vi "Change Steering Type.vi"(8 "error in (no error)":errorcluster, 10 "steering type":T1 items=["User Defined", "Differential", "Ackermann", "Mecanum"], 11 "dialog info in":T2={"steering frame ref"=refnum, "active wheel indexes"=[], "FP Refs"={"VI Refnum"=refnum, "Menu Ref"=refnum, "Sub Panel"=refnum, "picture"=refnum, "Steering Type"=refnum, "zoom in"=refnum, "zoom out"=refnum, "zoom extents"=refnum, "Wheels"=refnum, "Add Wheel"=refnum, "Remove Wheel"=refnum, "Copy Wheel"=refnum, "Angle Units"=refnum}, "subpanel info"={"subpanel VI refs"=[], "subpanel types"=[], "main to subpanel command events"=[]}, "picture dragging state"={"dragging"=FALSE, "wheel index"=-1, "dragging mode"=enum."translate", "wheel start position"={"x"=0.0, "y"=0.0, "theta"=0.0}, "relative mouse position"={"x"=0.0, "y"=0.0}, "relative mouse init angle (rad)"=0.0}, "picture size (pixels)"={"Width"=500, "Height"=500}, "picture grid"=bytes[0], "click zones group"={"click zones array"=[], "num click zones"=0}, "draw options"={"draw wheel states?"=FALSE, "highlight wheel index"=-1, "pixels per unit"=10.0, "draw forward velocity?"=FALSE, "velocity scale"=1.0}}) -> (0 "error out":errorcluster, 3 "dialog info out":T2={"steering frame ref"=refnum, "active wheel indexes"=[], "FP Refs"={"VI Refnum"=refnum, "Menu Ref"=refnum, "Sub Panel"=refnum, "picture"=refnum, "Steering Type"=refnum, "zoom in"=refnum, "zoom out"=refnum, "zoom extents"=refnum, "Wheels"=refnum, "Add Wheel"=refnum, "Remove Wheel"=refnum, "Copy Wheel"=refnum, "Angle Units"=refnum}, "subpanel info"={"subpanel VI refs"=[], "subpanel types"=[], "main to subpanel command events"=[]}, "picture dragging state"={"dragging"=FALSE, "wheel index"=-1, "dragging mode"=enum."translate", "wheel start position"={"x"=0.0, "y"=0.0, "theta"=0.0}, "relative mouse position"={"x"=0.0, "y"=0.0}, "relative mouse init angle (rad)"=0.0}, "picture size (pixels)"={"Width"=500, "Height"=500}, "picture grid"=bytes[0], "click zones group"={"click zones array"=[], "num click zones"=0}, "draw options"={"draw wheel states?"=FALSE, "highlight wheel index"=-1, "pixels per unit"=10.0, "draw forward velocity?"=FALSE, "velocity scale"=1.0}})   [LabVIEW 2017, in "NI_Robotics_Configure Steering Frame.lvlib"]
uses:
  <vilib>/robotics/Dialog/Configure Steering Frame/NI_Robotics_Configure Steering Frame.lvlib
  <vilib>/robotics/Dialog/Configure Steering Frame/Dialog Info.ctl
  <vilib>/robotics/Steering/Steering Frame/NI_Robotics_Steering Frame.lvclass
  <vilib>/robotics/Dialog/Configure Steering Frame/FP Refs.ctl
  <vilib>/robotics/Dialog/Configure Steering Frame/Subpanel Info.ctl
  <vilib>/robotics/Dialog/Configure Steering Frame/Main to Subpanel Command Event.ctl
  <vilib>/robotics/Dialog/Configure Steering Frame/Main to Subpanel Command.ctl
  <vilib>/robotics/Dialog/Configure Steering Frame/Dragging State.ctl
  <vilib>/robotics/Dialog/Configure Steering Frame/Dragging Mode.ctl
  <vilib>/Utility/miscctls.llb/LVBoundsTypeDef.ctl
  <vilib>/robotics/Dialog/Configure Steering Frame/Click Zone.ctl
  <vilib>/robotics/Utilities/Visualization/Steering Visualization/Steering Picture/Draw Steering Frame Options.ctl
  <vilib>/robotics/Dialog/Configure Steering Frame/Steering Type.ctl
  <vilib>/robotics/Steering/Steering Frame/NI_Robotics_Steering Frame.lvclass/NI_Robotics_Steering Frame.ctl
  <vilib>/robotics/Steering/Steering Frame/Get Multiple Wheels in Steering Frame.vi
  <vilib>/robotics/Steering/Differential Steering Frame/NI_Robotics_Differential Steering Frame.lvclass
  c:/Program Files (x86)/National Instruments/LabVIEW 2017/vi.lib/robotics/Steering/Steering Frame/NI_Robotics_Steering Frame.lvclass
  <vilib>/robotics/Steering/Ackermann Steering Frame/NI_Robotics_Ackermann Steering Frame.lvclass
  <vilib>/robotics/Steering/Mecanum Steering Frame/NI_Robotics_Mecanum Steering Frame.lvclass
  <vilib>/robotics/Steering/Steering Frame/Create User Defined Steering Frame.vi
  <vilib>/robotics/Steering/Wheel/NI_Robotics_Wheel.lvclass
  <vilib>/robotics/Utilities/Visualization/Steering Visualization/Steering Picture/NI_Robotics_Steering Picture.lvlib
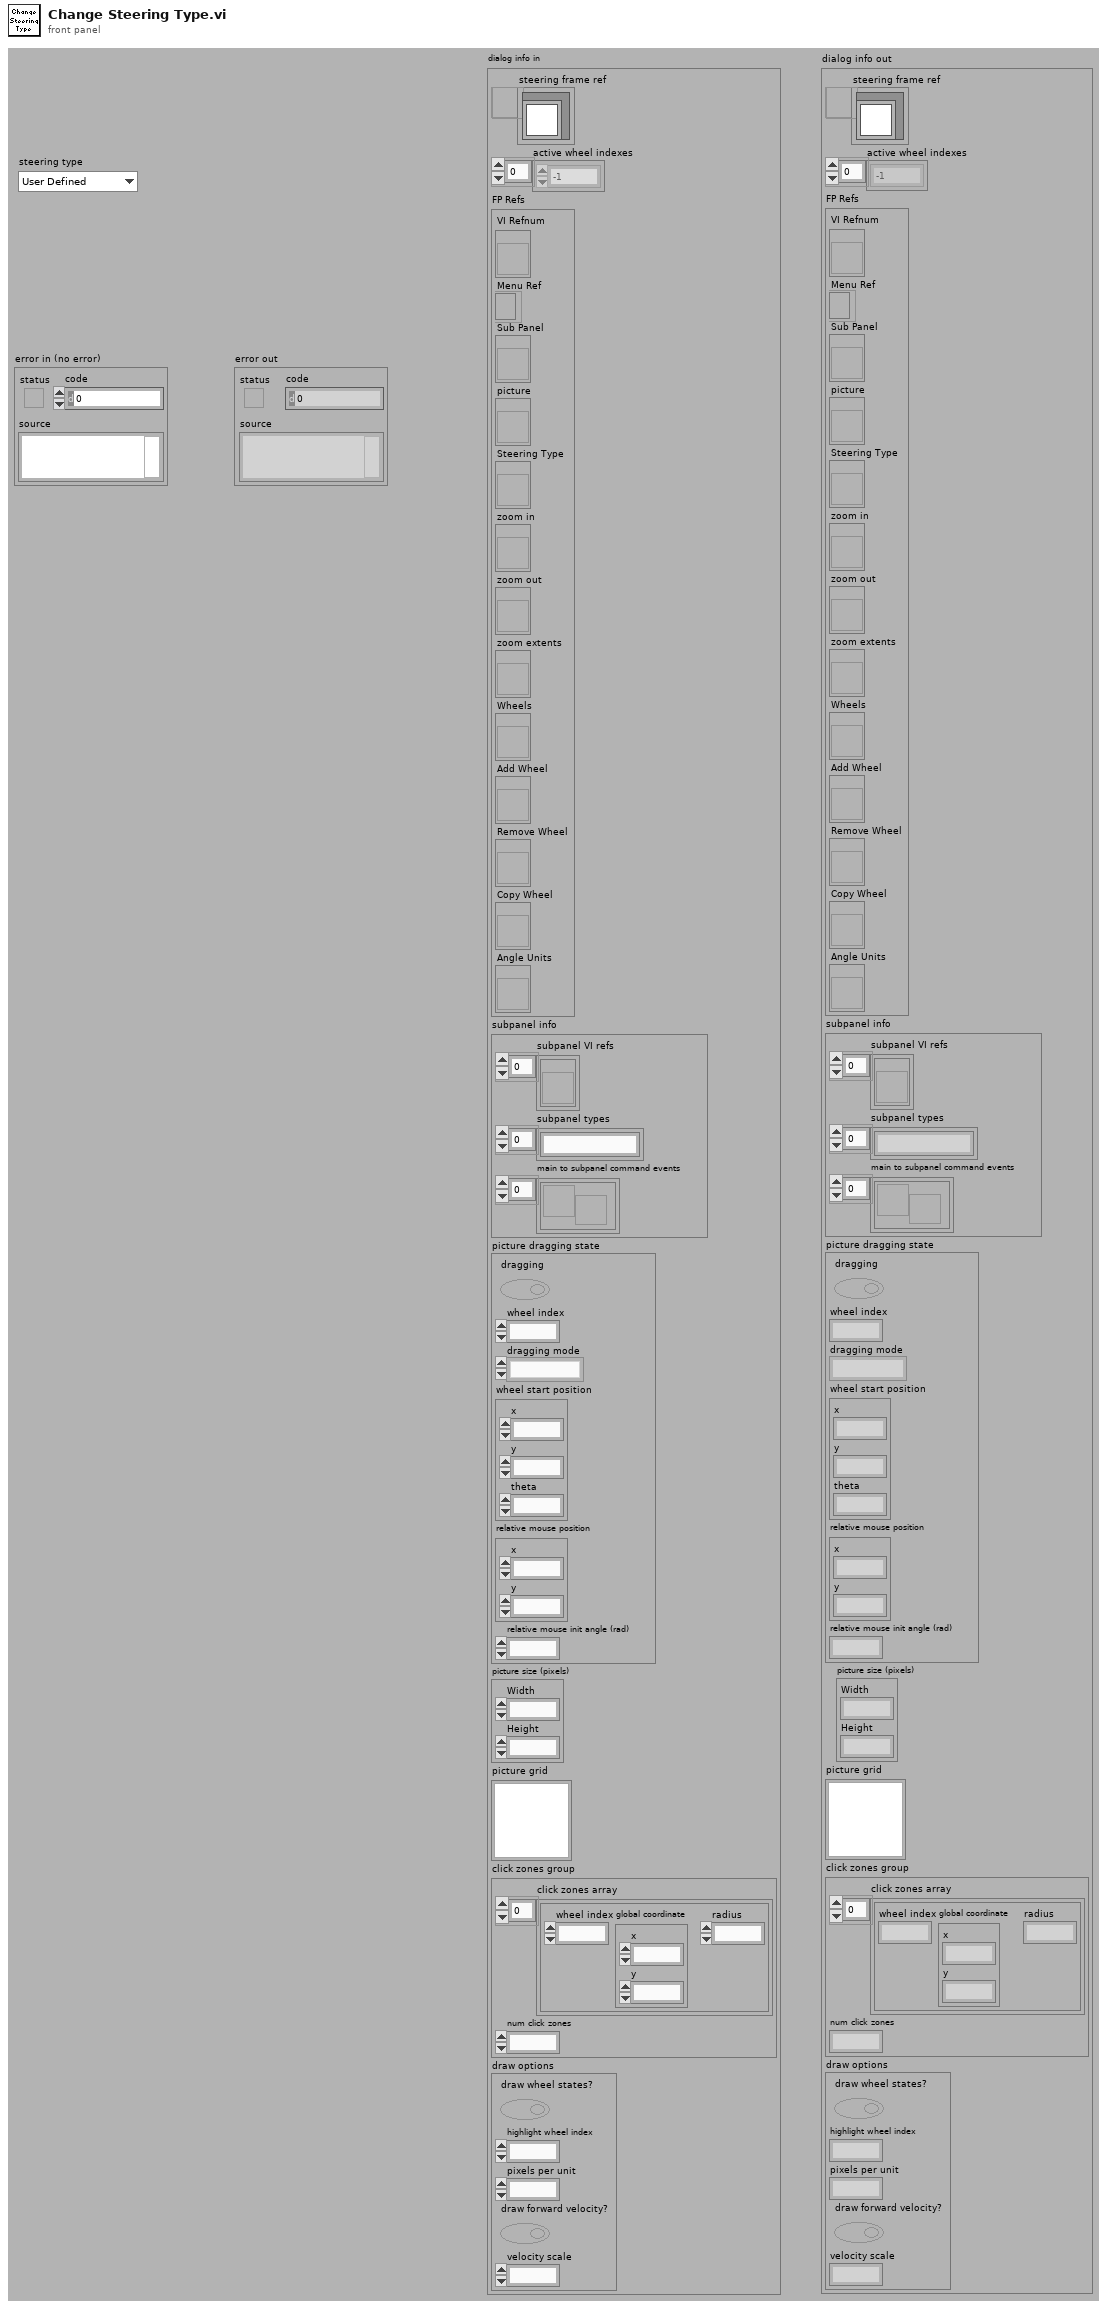
[diagram p1: front panel]
types:
  T1 = typedef "NI_Robotics_Configure Steering Frame.lvlib/Steering Type.ctl" = u16
  T2 = typedef "NI_Robotics_Configure Steering Frame.lvlib/Dialog Info.ctl" = cluster{"steering frame ref":refnum<data-value>, "active wheel indexes":i32[], "FP Refs":T3, "subpanel info":T4, "picture dragging state":T6, "picture size (pixels)":T8, "picture grid":picture, "click zones group":cluster{"click zones array":T9[], "num click zones":i32}, "draw options":T10}
  T3 = typedef "NI_Robotics_Configure Steering Frame.lvlib/FP Refs.ctl" = cluster{"VI Refnum":refnum<vi>, "Menu Ref":refnum<k9>, "Sub Panel":refnum<vi>, "picture":refnum<vi>, "Steering Type":refnum<vi>, "zoom in":refnum<vi>, "zoom out":refnum<vi>, "zoom extents":refnum<vi>, "Wheels":refnum<vi>, "Add Wheel":refnum<vi>, "Remove Wheel":refnum<vi>, "Copy Wheel":refnum<vi>, "Angle Units":refnum<vi>}
  T4 = typedef "NI_Robotics_Configure Steering Frame.lvlib/Subpanel Info.ctl" = cluster{"subpanel VI refs":refnum<vi>[], "subpanel types":string[], "main to subpanel command events":T5[]}
  T5 = typedef "NI_Robotics_Configure Steering Frame.lvlib/Main to Subpanel Command Event.ctl" = refnum<user-event>
  T6 = typedef "NI_Robotics_Configure Steering Frame.lvlib/Dragging State.ctl" = cluster{"dragging":bool, "wheel index":i32, "dragging mode":T7, "wheel start position":cluster{"x":dbl, "y":dbl, "theta":dbl}, "relative mouse position":cluster{"x":dbl, "y":dbl}, "relative mouse init angle (rad)":dbl}
  T7 = typedef "NI_Robotics_Configure Steering Frame.lvlib/Dragging Mode.ctl" = enum16{"translate", "rotate"}
  T8 = typedef "LVBoundsTypeDef.ctl" = cluster{"Width":u32, "Height":u32}
  T9 = typedef "NI_Robotics_Configure Steering Frame.lvlib/Click Zone.ctl" = cluster{"wheel index":i32, "global coordinate":cluster{"x":dbl, "y":dbl}, "radius":dbl}
  T10 = typedef "NI_Robotics_Steering Picture.lvlib/Draw Steering Frame Options.ctl" = cluster{"draw wheel states?":bool, "highlight wheel index":i32, "pixels per unit":dbl, "draw forward velocity?":bool, "velocity scale":dbl}
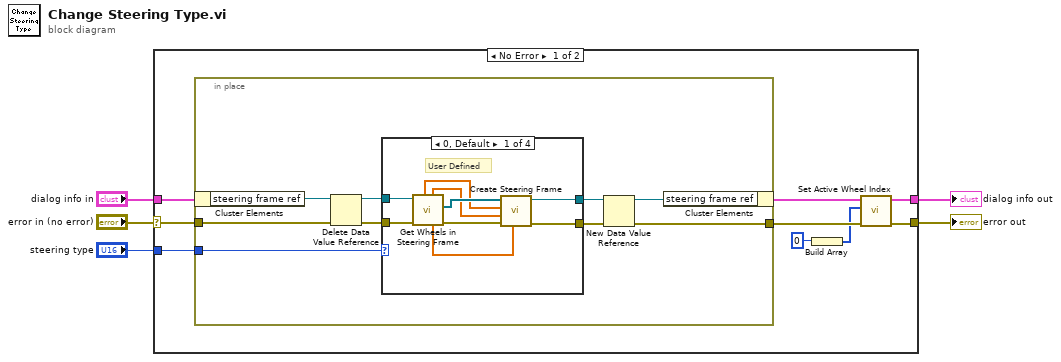
[diagram p0: block diagram]
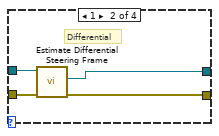
[diagram p2: hidden frame]
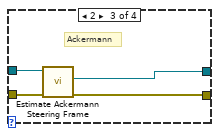
[diagram p3: hidden frame]
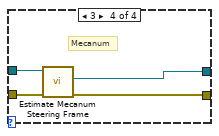
[diagram p4: hidden frame]
diagram:
  n1 = case shown="No Error" "error in (no error)" {
    selector: "error in (no error)" -> [w14 w46]
    tunnel: [w9 w46] -> w4
    tunnel: "dialog info in" -> [w12 w45]
    tunnel: [w10 w45] -> w2
    tunnel: "steering type" -> [w13 _]
    frame No Error {
      n2 = in-place {
        in-place-border: w14 -> [w22]
        in-place-border: w13 -> [w23]
        in-place-border: [w17] -> w8
        n3 = in-place-cluster #1(w12) -> ("steering frame ref"=w19:refnum<data-value>)
        n4 = Delete Data Value Reference(data value reference=w19, error in=w22) -> (data value=w20:refnum<class "NI_Robotics_Steering Frame.lvclass">, error out=w21:errorcluster)
        n5 = case shown="0, Default" w23 {
          tunnel: w21 -> [w31 w36 w37 w41]
          tunnel: w20 -> [w32 w34 w39 w42]
          tunnel: [w25 w33 w40 w44] -> w18
          tunnel: [w24 w35 w38 w43] -> w15
          frame 0, Default {
            # "User Defined"
            n6 = call-poly <vilib>:"Get Wheels in Steering Frame.vi"("error in (no error)"=w31, "steering frame in"=w32) -> ("error out"=w26:errorcluster, "wheels"=w30:refnum<class "NI_Robotics_Wheel.lvclass">[], "frame angles (rad)"=w27:dbl[], "y positions"=w28:dbl[], "x positions"=w29:dbl[])  [unwired: 3 in, 2 out]
            n7 = call-poly <vilib>:"Create Steering Frame.vi"("wheel frame angles (rad)"=w27, "error in (no error)"=w26, "wheel y positions"=w28, "wheel x positions"=w29, "wheels"=w30) -> ("error out"=w24:errorcluster, "steering frame out"=w25:refnum<class "NI_Robotics_Steering Frame.lvclass">)  [unwired: 5 in]
          }
          frame 1 {
            # "Differential"
            n8 = call <vilib>:"Estimate Differential Steering Frame.vi"("error in (no error)"=w36, "steering frame in"=w34) -> ("error out"=w35:errorcluster, "estimated differential steering frame copy"=w33:refnum<class "NI_Robotics_Differential Steering Frame.lvclass">)  [unwired: 7 in, 1 out]
          }
          frame 2 {
            # "Ackermann"
            n9 = call <vilib>:"Estimate Ackermann Steering Frame.vi"("error in (no error)"=w37, "steering frame in"=w39) -> ("error out"=w38:errorcluster, "estimated ackermann steering frame copy"=w40:refnum<class "NI_Robotics_Ackermann Steering Frame.lvclass">)  [unwired: 7 in, 1 out]
          }
          frame 3 {
            # "Mecanum"
            n10 = call <vilib>:"Estimate Mecanum Steering Frame.vi"("error in (no error)"=w41, "steering frame in"=w42) -> ("error out"=w43:errorcluster, "estimated mecanum steering frame copy"=w44:refnum<class "NI_Robotics_Mecanum Steering Frame.lvclass">)  [unwired: 7 in, 1 out]
          }
        }
        n11 = New Data Value Reference(data value=w18, error in=w15) -> (data value reference=w16:refnum<data-value>, error out=w17:errorcluster)
        n12 = in-place-cluster #1("steering frame ref"=w16) -> (w11:T2)
      }
      n13 = Build Array(0) -> (w6:i32[])
      n14 = call <vilib>:"Set Active Wheel Index.vi"("error in (no error)"=w8, "active wheel indexes"=w6, "dialog info in"=w11) -> ("error out"=w9:errorcluster, "dialog info out"=w10:T2)  [unwired: 7 in]
    }
    frame Error {
    }
  }
  "error out" <- w4
  "dialog info out" <- w2
